vi "文件名（旧）.vi"(8 "第n个文件":i32, 9 "文件类型":i32) -> (2 "添加的路径":path)   [LabVIEW 2018]
uses:
  <vilib>/Utility/sysdir.llb/System Directory Type.ctl
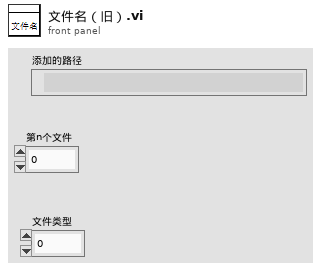
[diagram p1: front panel]
types:
  T1 = typedef "System Directory Type.ctl" = i32
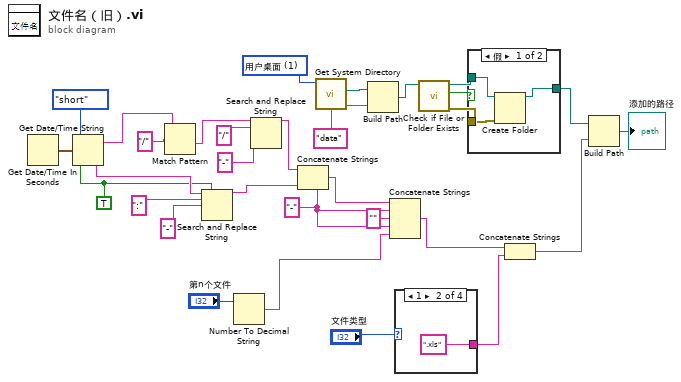
[diagram p0: block diagram]
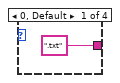
[diagram p2: hidden frame]
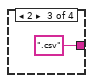
[diagram p3: hidden frame]
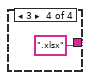
[diagram p4: hidden frame]
diagram:
  w5 = TRUE ("需要秒？(F)")
  w19 = "-" ("字符串")
  w27 = T1 1 items=["用户目录"=0, "用户桌面"=1, "用户文档"=2, "用户应用程序数据"=3, "用户设置"=4, "用户临时目录"=5, "公共文档"=6, "公共应用程序数据"=7, "公共设置"=8, "公共缓存"=13, "系统核心库"=9, "系统安装库"=10, "应用程序文件"=11, "启动盘根目录"=12] ("system directory type")
  n1 = Get Date/Time In Seconds() -> (seconds since 1Jan1904=w31:timestamp)
  n2 = Get Date/Time String(date format (0)=enum16{"short", "long", "abbreviated"}."short" ("日期格式(0)"), seconds (now)=w31, want seconds? (F)=w5) -> (date string=w29:string, time string=w14:string)
  n3 = Match Pattern(string=w29, regular expression="/" ("正则表达式")) -> (after substring=w18:string)  [unwired: 1 in, 3 out]
  n4 = Search and Replace String(replace all?=w5, input string=w14, search string=":" ("搜索字符串"), replace string="-" ("替换字符串(\"\")")) -> (result string=w11:string)  [unwired: 4 in, 3 out]
  n5 = Number To Decimal String(number="第n个文件") -> (decimal integer string=w4:string)  [unwired: 1 in]
  n6 = Search and Replace String(input string=w18, search string="/" ("搜索字符串"), replace string="-" ("替换字符串(\"\")")) -> (result string=w16:string)  [unwired: 5 in, 3 out]
  n7 = Concatenate Strings(w16, w19, w11) -> (w21:string)
  n8 = call <vilib>:"Get System Directory.vi"("system directory type"=w27) -> ("system directory"=w26:path)  [unwired: 10 in]
  n9 = Build Path(base path=w26, name or relative path="data" ("名称或相对路径")) -> (appended path=w10:path)
  n10 = Concatenate Strings(w21, w19, "" ("字符串"), w19, w4) -> (w23:string)
  n11 = case shown="1" "文件类型" {
    tunnel: [".txt" ".xls" ".csv" ".xlsx"] -> w3
    frame 0, Default {
    }
    frame 1 {
    }
    frame 2 {
    }
    frame 3 {
    }
  }
  n12 = call <vilib>:"Check if File or Folder Exists.vi"("path"=w10) -> ("error out"=w6:errorcluster, "file or folder exists?"=w9:bool, "dup path"=w7:path)  [unwired: 8 in]
  n13 = case shown="假" w9 {
    tunnel: [w38 w39] -> w8
    tunnel: w7 -> [w37 w39]
    tunnel: w6 -> [w36 _]
    frame False {
      n14 = Create Folder(path (use dialog)=w37, error in=w36) -> (created path=w38:path)  [unwired: 1 in, 2 out]
    }
    frame True {
    }
  }
  n15 = Concatenate Strings(w23, w3) -> (w22:string)
  n16 = Build Path(base path=w8, name or relative path=w22) -> (appended path=→"添加的路径":path)
